vi "loadCellControl.vi"() -> ()   [LabVIEW 2013]
panel:
  in  "Tab Control":enum32{"Formatted Data", "Raw Data"}(tab)
  out "Saved to:":path
  out "Lbs (Average)":dbl
  out "Scaled":dynamicdata(graph)
  in  "Volt-Lbs Zero":dbl
  in  "Volts-Lbs coeff.":dbl=150.0
  out "Scaled 2":dynamicdata(graph)
  out "Raw Data":dynamicdata(graph)
  out "Raw Data 2":dynamicdata(graph)
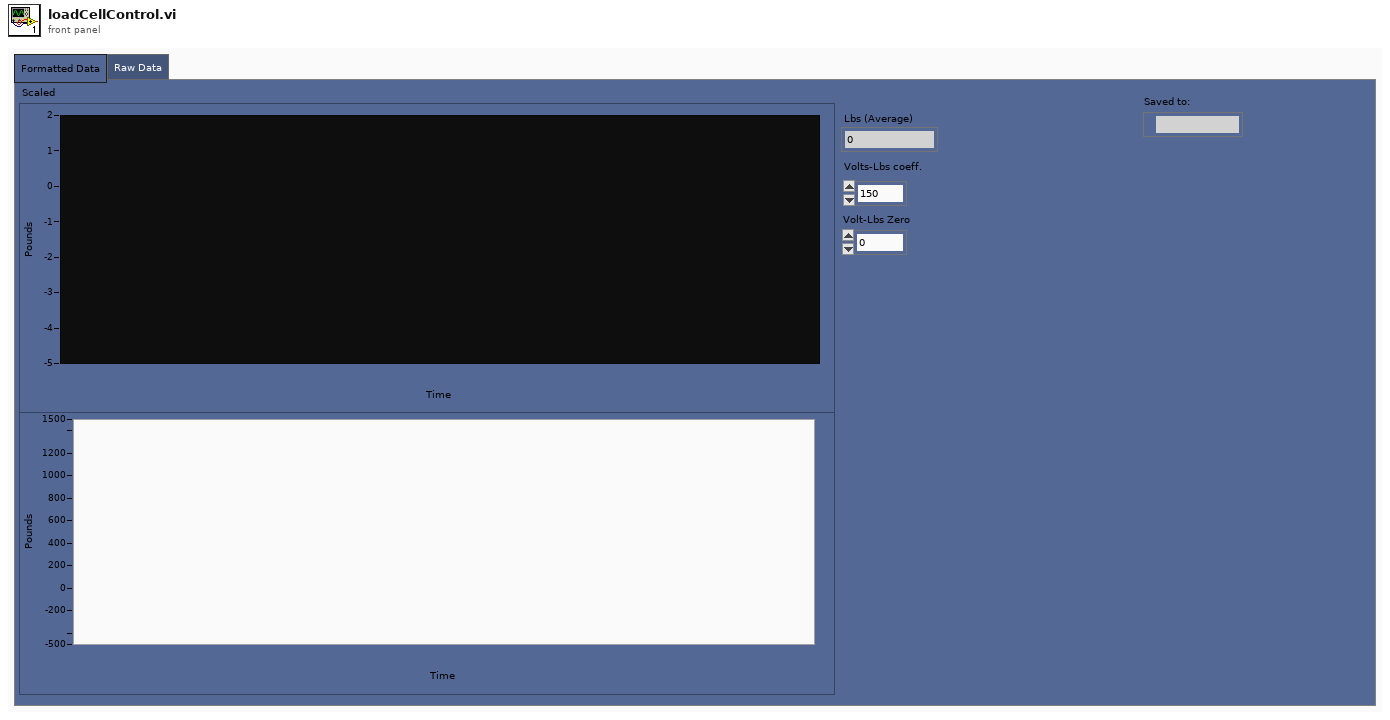
[diagram p1: front panel]
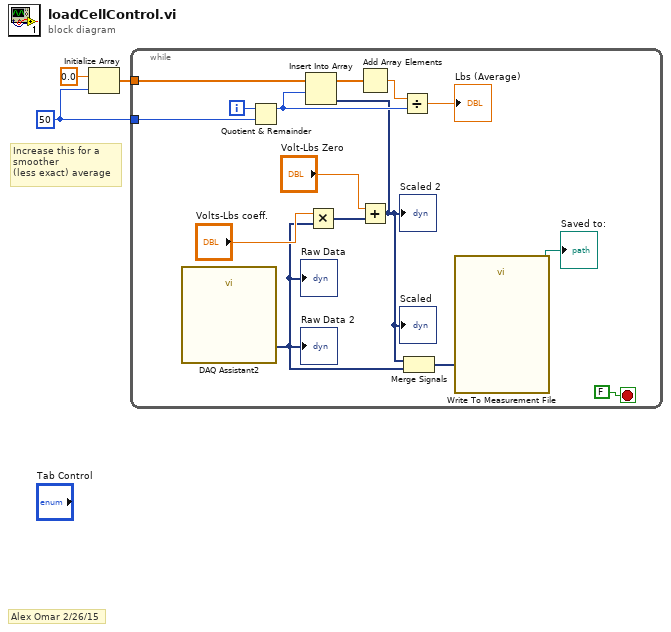
[diagram p0: block diagram]
diagram:
  w1 = 50
  # "Alex Omar 2/26/15"
  # "Increase this for a smoother\n(less exact) average"
  n1 = Initialize Array(0.0, w1) -> (w3:dbl[])
  n2 = while {
    tunnel: w3 -> [w16]
    tunnel: w1 -> [w15]
    i -> [w14]
    stop <- FALSE stop-if-true
    n3 = call "DAQ Assistant2"() -> ("data"=w8:dynamicdata)  [unwired: 16 in, 3 out]
    "Raw Data" <- w8
    "Raw Data 2" <- w8
    n4 = Quotient & Remainder(x=w14, y=w15) -> (x-y*floor(x/y)=w11:i32)  [unwired: 1 out]
    n5 = Multiply(x="Volts-Lbs coeff.", y=w8) -> (x*y=w7:dynamicdata)
    n6 = Add(x="Volt-Lbs Zero", y=w7) -> (x+y=w4:dynamicdata)
    "Scaled" <- w4
    "Scaled 2" <- w4
    n7 = Insert Into Array(array=w16, index=w11, new element=w4) -> (w13:dbl[])
    n8 = Add Array Elements(numeric array=w13) -> (sum=w12:dbl)
    n9 = Divide(x=w12, y=w11) -> (x/y=→"Lbs (Average)":dbl)
    n10 = Merge Signals(w4, w8) -> (w9:dynamicdata)
    n11 = call "Write To Measurement File"("Signals"=w9) -> ("Filename Out"=→"Saved to:":path)  [unwired: 16 in, 2 out]
  }
